vi "PH_BlackBox.PC Move.vi"(0 "i ref in":refnum<vi>, 2 "Move?":bool, 5 "error in (no error)":errorcluster) -> (14 "i ref out":refnum<vi>, 19 "error out":errorcluster)   [LabVIEW 2014, in "PH_BlackBox.lvlib"]
doc: "Thi is the action done in the event case \"Move\"."
uses:
  PH_BlackBox.lvlib
  PH_Devices/PH_Beckhoff_Common/PH_Beckhoff_Common.lvlib
  PH_Devices/PH_Beckhoff/PH_Beckhoff.lvlib
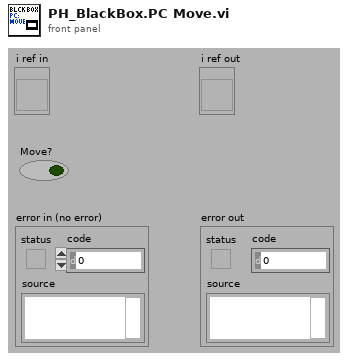
[diagram p1: front panel]
types:
  T1 = typedef "PH_BlackBox.lvlib/PH_BlackBox.i attribute.ctl" = cluster{"BB Remote Controlled?":bool, "GUI Refs":T2, "Position IN":T3, "Position OUT":T3, "BB Remote Controlled by other Instance?":bool, "Recipient":string, "Number":i32, "Caption Move":string, "Caption Out":string, "Caption In":string}
  T2 = typedef "PH_BlackBox.lvlib/PH_BlackBox.GUI Refs.ctl" = cluster{"MOVE IN":refnum<vi>, "MOVE":refnum<vi>, "IN":refnum<vi>, "OUT":refnum<vi>, "REMOTE":refnum<vi>, "GUI-Knob Move":refnum<vi>, "GUI-Knob Move in":refnum<vi>, "POWER ON":refnum<vi>, "Delete":refnum<vi>, "Function Textfield":refnum<vi>}
  T3 = typedef "PH_StatusHandler.lvlib/PH_StatusHandler.Status.ctl" = i16
  T4 = typedef "PH_Beckhoff_Common.lvlib/PH_Beckhoff_Common.BB Tagnames.ctl" = cluster{"Sensor Remote controlled":string, "Sensor Out":string, "Sensor In":string, "Actor Direction In":string, "Actor Move":string, "Sensor Power ok":string, "Instance":string}
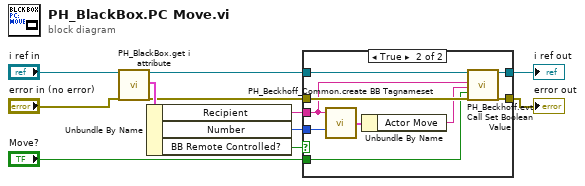
[diagram p0: block diagram]
diagram:
  n1 = call "PH_BlackBox.get i attribute.vi"("i ref in"="i ref in", "error in (no error)"="error in (no error)") -> ("i ref out"=w2:refnum<vi>, "i attribute"=w10:T1, "error out"=w1:errorcluster)  [unwired: 15 in]
  n2 = Unbundle By Name(w10) -> ("Recipient"=w3:string, "Number"=w4:i32, "BB Remote Controlled?"=w11:bool)
  n3 = case shown="True" w11 {
    tunnel: [w13 w19] -> w5
    tunnel: [w12 w20] -> w6
    tunnel: w2 -> [w13 w21]
    tunnel: w1 -> [w12 w22]
    tunnel: "Move?" -> [_ w18]
    tunnel: w4 -> [_ w17]
    tunnel: w3 -> [_ w15]
    frame False {
    }
    frame True {
      n4 = call "PH_Beckhoff_Common.create BB Tagnameset.vi"("#"=w17, "Instance Name"=w15) -> ("output cluster"=w16:T4)
      n5 = Unbundle By Name(w16) -> ("Actor Move"=w14:string)
      n6 = call "PH_Beckhoff.evt Call Set Boolean Value.vi"("i ref in"=w21, "Beckhoff Instance"=w15, "Tagname to set"=w14, "Value"=w18, "error in"=w22) -> ("i ref out"=w19:refnum<vi>, "error out"=w20:errorcluster)  [unwired: 13 in]
    }
  }
  "error out" <- w6
  "i ref out" <- w5
